vi "ACDC_Config_9234.vi"(8 "error in (no error)":errorcluster, 9 "Input Config Array":T1[](array[typedef])=[0, 0, 0, 0, 0, 0, 0, 0, 0, 0, 0, 0, 0, 0, 0, 0, 0, 0, 0, 0, 0, 0, 0, 0, 0, 0, 0, 0, 0, 0, 0, 0] items=["AC Coupled", "DC Coupled", "IEPE AC Coupled"], 10 "Data Rate [S/s]":u32) -> (0 "error out":errorcluster)   [LabVIEW 2017, in "BOP_VibAPI_2.lvlib"]
uses:
  <vilib>/addons/InsightCM/Devices/Shared/Cms/Fpga/Acquisition/source/subVIs/VibAPI_2/BOP_VibAPI_2.lvlib
  <vilib>/LabVIEW Targets/FPGA/cRIO/shared/nicrio_ModuleControls/nicrio_cRIO-9232_ConfigModeRing.ctl
  <vilib>/rvi/eio/common/nirviEmuTemplatePropertySet_errors.vi
  <vilib>/eio/EIOPropertyNode/EIOPropertyNode.xnode
  <vilib>/LabVIEW Targets/FPGA/cRIO/shared/nicrio_ModuleControls/nicrio_cRIO-9234_DataRatesRing2.ctl
  <vilib>/LabVIEW Targets/FPGA/cRIO/shared/nicrio_ModuleControls/nicrio_cRIO-9234_ConfigModeRing.ctl
  <vilib>/rvi/eio/common/nirviEmuTemplatePropertyGet_errors.vi
  <vilib>/rvi/eio/common/nirviEmuTemplatePropertyGet_noerrors.vi
  <vilib>/rvi/eio/common/nirviEmuTemplatePropertySet_noerrors.vi
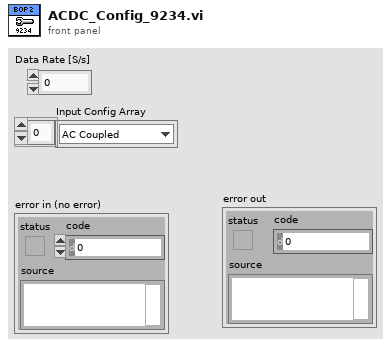
[diagram p1: front panel]
types:
  T1 = typedef "nicrio_cRIO-9232_ConfigModeRing.ctl" = u8
  T2 = typedef "nicrio_cRIO-9234_DataRatesRing2.ctl" = u8
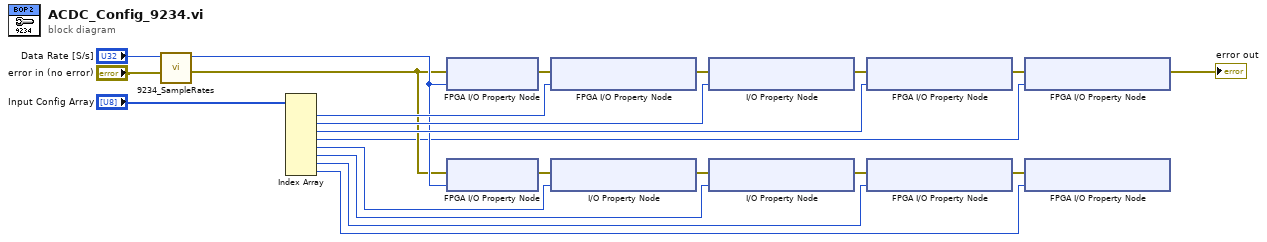
[diagram p0: block diagram]
diagram:
  n1 = call <vilib>:"9234_SampleRates.vi"("error in (no error)"="error in (no error)", "Data Rate [S/s]"="Data Rate [S/s]") -> ("error out"=w10:errorcluster, "Data Rate"=w11:T2)  [unwired: 8 in]
  n2 = Index Array(array="Input Config Array") -> (element #1=w14:T1, element #2=w13:T1, element #3=w12:T1, element #4=w2:T1, element #5=w3:T1, element #6=w4:T1, element #7=w6:T1, element #8=w1:T1)  [unwired: 8 in]
  n3 = xnode "FPGA I/O Property Node"("error in"=w10, "Data Rate"=w11) -> ("error out"=w16:errorcluster)  [unwired: 1 in, 1 out]
  n4 = xnode "FPGA I/O Property Node"("error in"=w10, "Data Rate"=w11) -> ("error out"=w15:errorcluster)  [unwired: 1 in, 1 out]
  n5 = xnode "FPGA I/O Property Node"("error in"=w16, "Input Configuration"=w14) -> ("error out"=w17:errorcluster)  [unwired: 1 in, 1 out]
  n6 = xnode "I/O Property Node"("error in"=w15, "Input Configuration"=w3) -> ("error out"=w19:errorcluster)  [unwired: 1 in, 1 out]
  n7 = xnode "I/O Property Node"("error in"=w17, "Input Configuration"=w13) -> ("error out"=w18:errorcluster)  [unwired: 1 in, 1 out]
  n8 = xnode "I/O Property Node"("error in"=w19, "Input Configuration"=w4) -> ("error out"=w20:errorcluster)  [unwired: 1 in, 1 out]
  n9 = xnode "FPGA I/O Property Node"("error in"=w18, "Input Configuration"=w12) -> ("error out"=w8:errorcluster)  [unwired: 1 in, 1 out]
  n10 = xnode "FPGA I/O Property Node"("error in"=w20, "Input Configuration"=w6) -> ("error out"=w5:errorcluster)  [unwired: 1 in, 1 out]
  n11 = xnode "FPGA I/O Property Node"("error in"=w8, "Input Configuration"=w2) -> ("error out"=→"error out":errorcluster)  [unwired: 1 in, 1 out]
  n12 = xnode "FPGA I/O Property Node"("error in"=w5, "Input Configuration"=w1) -> ()  [unwired: 1 in, 2 out]
